vi "Mandelbrot.vi"() -> ()   [LabVIEW 2011]
doc: "This VI will create a mandelbrot fractal image. You can modify the colors by changing the map in the color map section. In addition, you can also modify the depth and color scheme by changing the iteration maximum (currently set to 50)."
uses:
  <vilib>/Utility/miscctls.llb/LVBoundsTypeDef.ctl
  <vilib>/Analysis/1siggen.llb/Ramp Pattern by Samples.vi
  <vilib>/gmath/interp.llb/Create Mesh Grid (2D) (x,y arrays).vi
  <vilib>/Analysis/NI_AALBase.lvlib
  <vilib>/gmath/NI_Gmath.lvlib
panel:
  in  "Iterations":u32=200
  in  "Resolution":u32=1000
  out "Horizontal Graduated Bar":dbl(slide) scale=0.0..1.0
  in  "Reset":bool
  in  "Redraw":bool
  in  "stop":bool
  in  "Im_min":dbl=-0.2692643193522379
  in  "Im_max":dbl=-0.2692638610655374
  in  "Re_min":dbl=-0.9020780585133482
  in  "Re_max":dbl=-0.9020777170269695
  out "Intensity Graph":u32[][](graph)
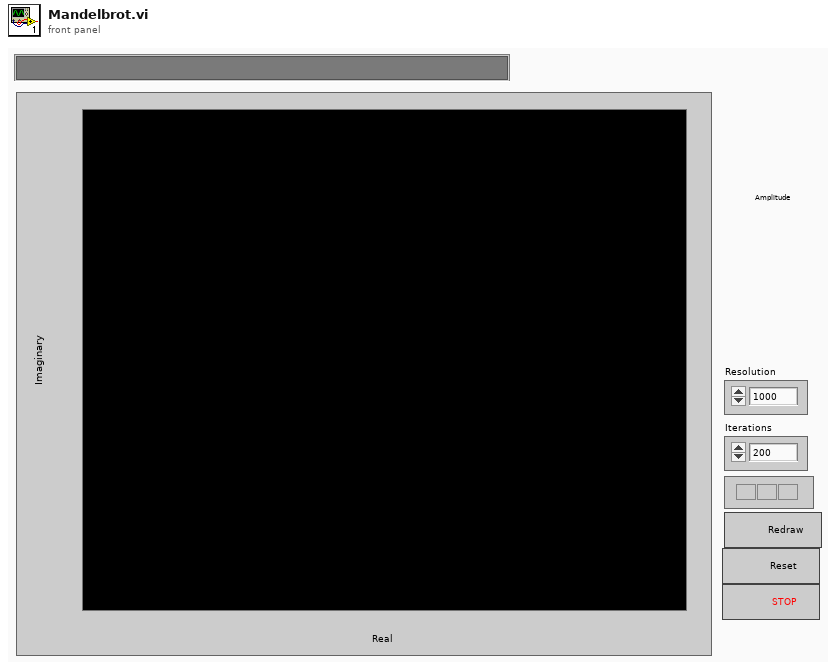
[diagram p1: front panel]
types:
  T1 = typedef "LVBoundsTypeDef.ctl" = cluster{"Width":u32, "Height":u32}
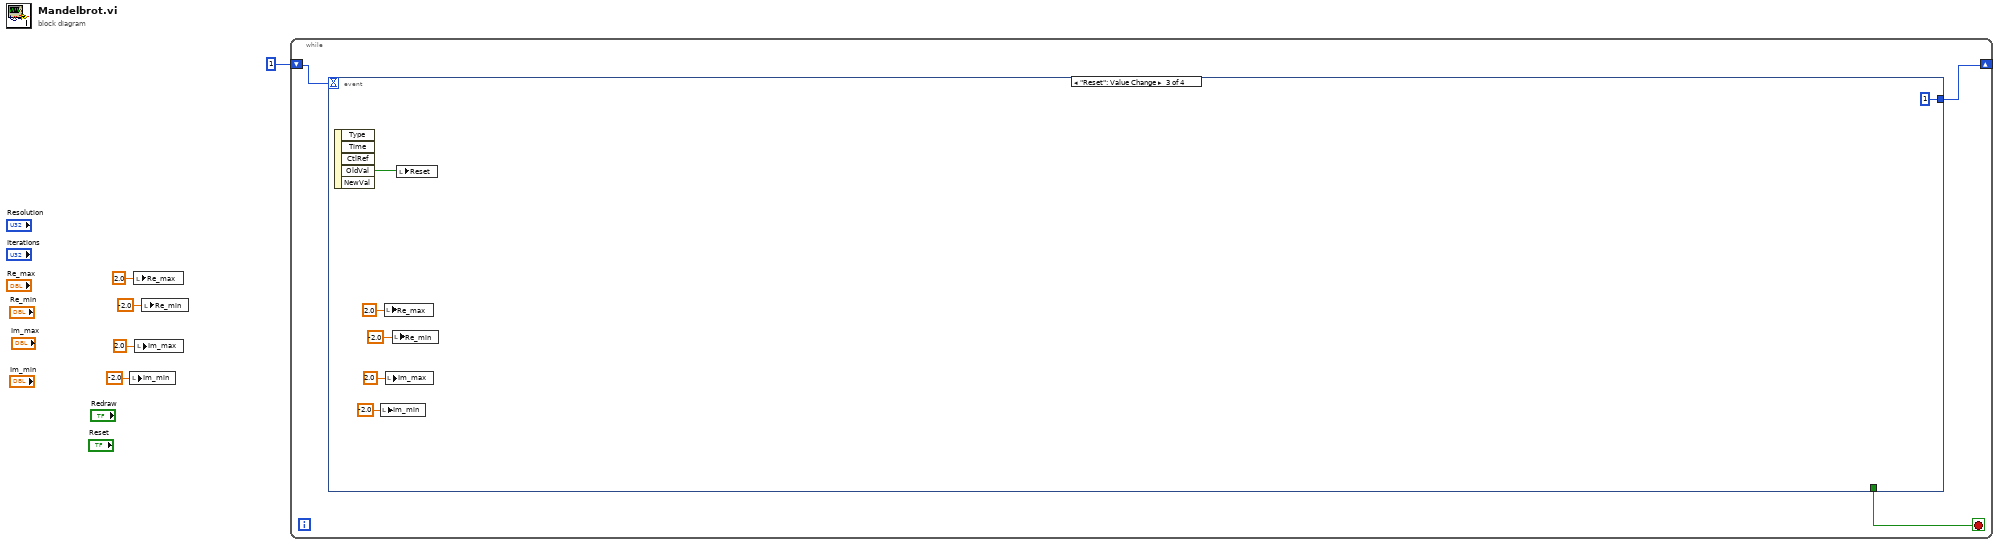
[diagram p0: block diagram]
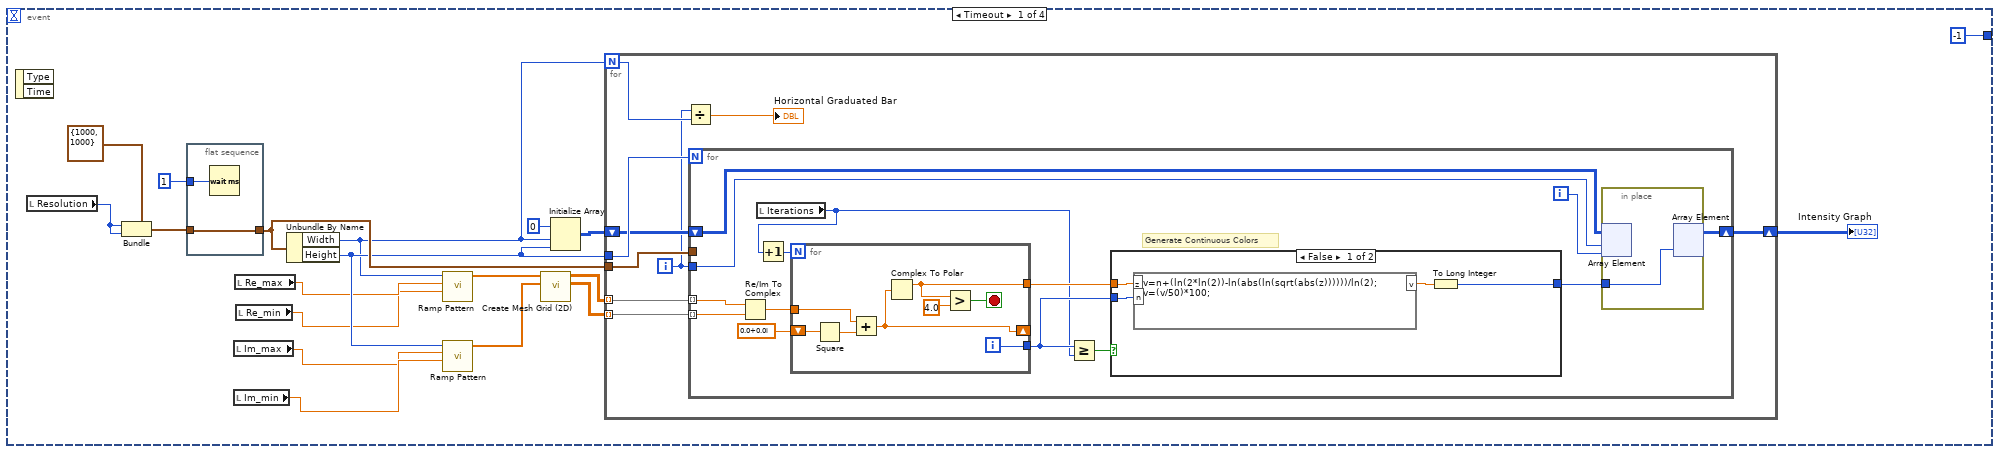
[diagram p2: hidden frame]
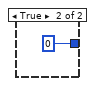
[diagram p3: hidden frame]
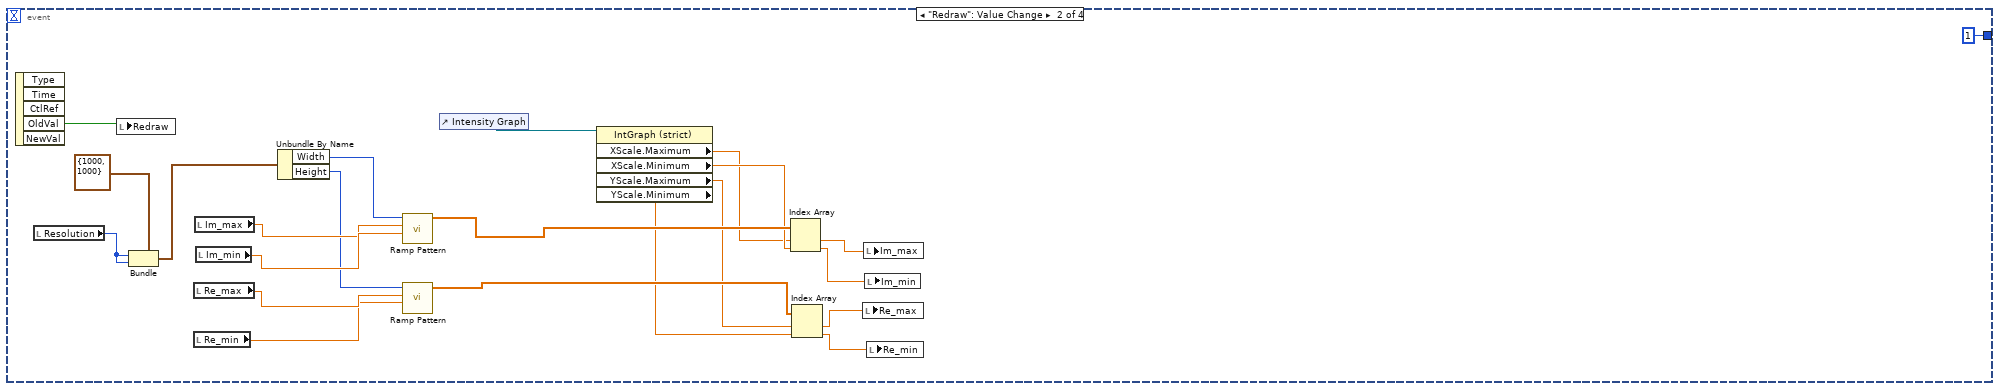
[diagram p4: hidden frame]
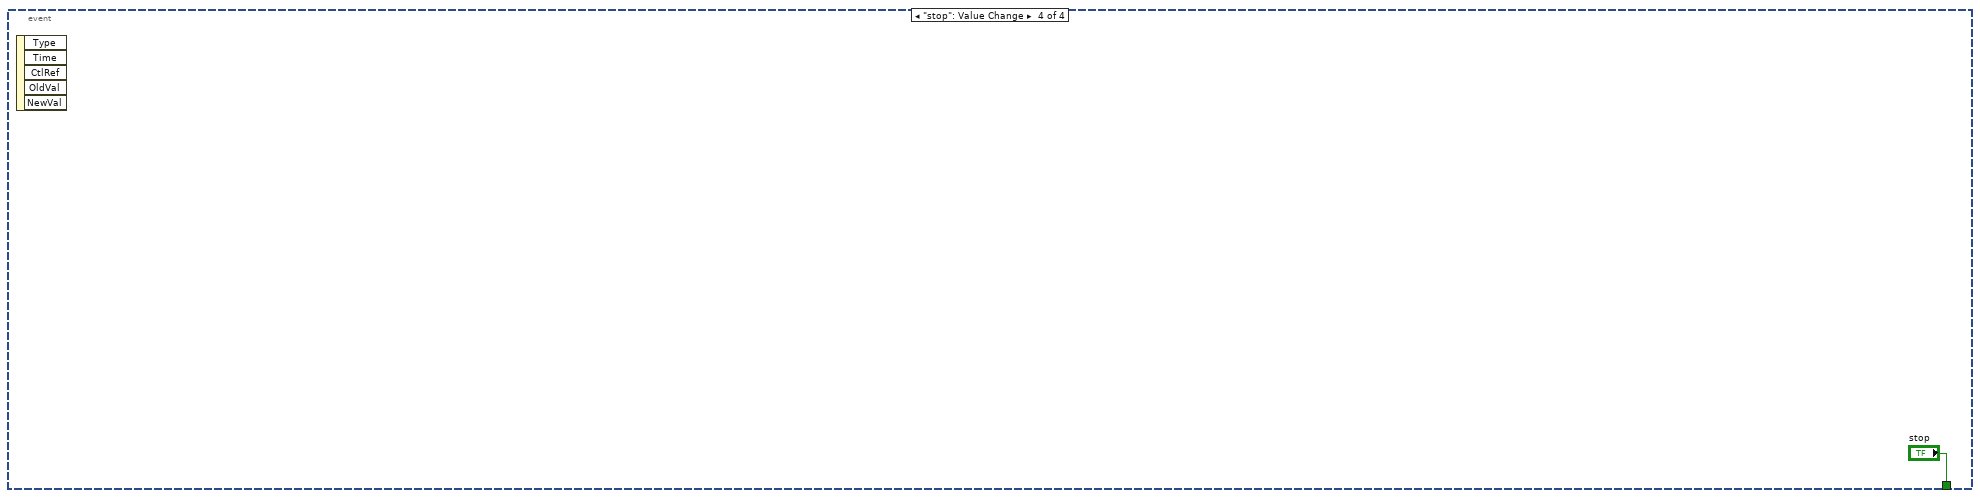
[diagram p5: hidden frame]
diagram:
  n1 = local write "Im_min"(-2.0 ("Im_min")) -> ()
  n2 = local write "Re_max"(2.0 ("Re_max")) -> ()
  n3 = local write "Im_max"(2.0 ("Im_max")) -> ()
  n4 = local write "Re_min"(-2.0 ("Re_min")) -> ()
  n5 = while {
    shift-right: [w7] -> _
    shift-left: 1 -> [w8]
    stop <- w6 stop-if-true
    n6 = event shown="[2] \"Reset\": Value Change" {
      selector: _ -> [_ _ _ _]
      dyn-events: _ -> [_ _ _ _]
      timeout: w8 -> [_ _ _ _]
      tunnel: [-1 1 1 _] -> w7
      tunnel: [_ _ _ "stop"] -> w6
      event Timeout {
        n7 = event-data() -> ()  [unwired: 1 in, 2 out]
        n8 = local read "Resolution"() -> (w9:u32)
        n9 = Bundle(cluster=T1 {"Width"=1000, "Height"=1000} ("Draw Area Size"), "Width"=w9, "Height"=w9) -> (w10:T1)
        n10 = flat-sequence {
          tunnel: w10 -> [w29]
          tunnel: [w29] -> w27
          tunnel: u32 1 ("milliseconds to wait") -> [w28]
          frame #0 {
            n11 = Wait (ms)(milliseconds to wait=w28) -> ()  [unwired: 1 out]
          }
        }
        n12 = local read "Im_max"() -> (w14:dbl)
        n13 = local read "Im_min"() -> (w15:dbl)
        n14 = local read "Re_max"() -> (w16:dbl)
        n15 = local read "Re_min"() -> (w13:dbl)
        n16 = Unbundle By Name(w27) -> ("Width"=w21:u32, "Height"=w22:u32)
        n17 = call-poly <vilib>:"Ramp Pattern.vi"("start"=w13, "end"=w16, "samples"=w21) -> ("Ramp Pattern"=w20:dbl[])  [unwired: 7 in, 1 out]
        n18 = call-poly <vilib>:"Ramp Pattern.vi"("start"=w15, "end"=w14, "samples"=w22) -> ("Ramp Pattern"=w19:dbl[])  [unwired: 7 in, 1 out]
        n19 = call-poly <vilib>:"Create Mesh Grid (2D).vi"("y domain"=w19, "x domain"=w20) -> ("Y"=w17:dbl[][], "X"=w18:dbl[][])  [unwired: 7 in, 1 out]
        n20 = Initialize Array(u32 0 ("element"), w21, w22) -> (w25:u32[][])
        n21 = for {
          N: w21 -> [w32]
          tunnel: w22 -> [w38]
          tunnel: w27 -> [w37]
          shift-right: [w35] -> w24
          shift-left: w25 -> [w36]
          tunnel: w18 -> [w34] mode=indexing
          tunnel: w17 -> [w33] mode=indexing
          i -> [w31]
          n22 = Divide(x=w31, y=w32) -> (x/y=→"Horizontal Graduated Bar":dbl)
          n23 = for {
            N: w38 -> [_]
            tunnel: w31 -> [w47]
            tunnel: w37 -> [_]
            shift-right: [w48] -> w35
            shift-left: w36 -> [w49]
            tunnel: w34 -> [w42] mode=indexing
            tunnel: w33 -> [w41] mode=indexing
            i -> [w46]
            # "Generate Continuous Colors"
            n24 = Re/Im To Complex(1:w41, 2:w42) -> (0:w43:cdb)
            n25 = local read "Iterations"() -> (w40:u32)
            n26 = Increment(x=w40) -> (x+1=w39:u32)
            n27 = for {
              N: w39 -> [_]
              tunnel: w43 -> [w59]
              shift-right: [w57] -> _
              shift-left: cdb 0.0+0.0i ("x + iy") -> [w60]
              tunnel: [w54] -> w51
              tunnel: [w53] -> w50
              i -> [w53]
              stop <- w55 stop-if-true
              n28 = Square(x=w60) -> (x^2=w58:cdb)
              n29 = Add(x=w59, y=w58) -> (x+y=w57:cdb)
              n30 = Complex To Polar(r * e^(i*theta)=w57) -> (r=w54:dbl)  [unwired: 1 out]
              n31 = Greater?(x=w54, y=4.0) -> (0:w55:bool)
            }
            n32 = Greater Or Equal?(x=w50, y=w40) -> (x >= y?=w52:bool)
            n33 = case shown="False" w52 {
              tunnel: [w65 0] -> w45
              tunnel: w51 -> [w64 _]
              tunnel: w50 -> [w63 _]
              frame False {
                n34 = formula code="v=n+(ln(2*ln(2))-ln(abs(ln(sqrt(abs(z))))))/ln(2);\nv=(v/50)*100;"("z"=w64, "n"=w63) -> ("v"=w62:dbl)
                n35 = To Long Integer(number=w62) -> (32bit integer=w65:i32)
              }
              frame True {
              }
            }
            n36 = in-place {
              in-place-border: w45 -> [w61]
              n37 = in-place-array #1(w49, w47, w46) -> ()  [unwired: 1 out]
              n38 = in-place-array #1(w61) -> (w48:u32[][])  [unwired: 2 out]
            }
          }
        }
        "Intensity Graph" <- w24
      }
      event "Redraw": Value Change {
        n39 = event-data() -> ("OldVal"=w88:bool)  [unwired: 1 in, 4 out]
        n40 = local read "Resolution"() -> (w68:u32)
        n41 = local write "Redraw"(w88) -> ()
        n42 = Bundle(cluster=T1 {"Width"=1000, "Height"=1000} ("Draw Area Size"), "Width"=w68, "Height"=w68) -> (w67:T1)
        n43 = local read "Re_max"() -> (w85:dbl)
        n44 = local read "Re_min"() -> (w82:dbl)
        n45 = local read "Im_max"() -> (w84:dbl)
        n46 = local read "Im_min"() -> (w86:dbl)
        n47 = Unbundle By Name(w67) -> ("Width"=w81:u32, "Height"=w83:u32)
        n48 = call-poly <vilib>:"Ramp Pattern.vi"("start"=w86, "end"=w84, "samples"=w81) -> ("Ramp Pattern"=w79:dbl[])  [unwired: 7 in, 1 out]
        n49 = call-poly <vilib>:"Ramp Pattern.vi"("start"=w82, "end"=w85, "samples"=w83) -> ("Ramp Pattern"=w73:dbl[])  [unwired: 7 in, 1 out]
        n50 = control-ref of="Intensity Graph"() -> (w80:refnum<vi>)
        n51 = property class="IntGraph (strict)"(reference=w80) -> ("XScale.Maximum"=w70:dbl, "XScale.Minimum"=w77:dbl, "YScale.Maximum"=w72:dbl, "YScale.Minimum"=w71:dbl)  [unwired: 1 in, 2 out]
        n52 = Index Array(array=w79, index #1=w70, index #2=w77) -> (element #1=w78:dbl, element #2=w76:dbl)
        n53 = Index Array(array=w73, index #1=w72, index #2=w71) -> (element #1=w75:dbl, element #2=w74:dbl)
        n54 = local write "Re_max"(w75) -> ()
        n55 = local write "Im_max"(w78) -> ()
        n56 = local write "Im_min"(w76) -> ()
        n57 = local write "Re_min"(w74) -> ()
      }
      event "Reset": Value Change {
        n58 = event-data() -> ("OldVal"=w94:bool)  [unwired: 1 in, 4 out]
        n59 = local write "Im_min"(-2.0 ("Im_min")) -> ()
        n60 = local write "Re_max"(2.0 ("Re_max")) -> ()
        n61 = local write "Im_max"(2.0 ("Im_max")) -> ()
        n62 = local write "Re_min"(-2.0 ("Re_min")) -> ()
        n63 = local write "Reset"(w94) -> ()
      }
      event "stop": Value Change {
        n64 = event-data() -> ()  [unwired: 1 in, 5 out]
      }
    }
  }
